vi "setCenter.vi"(8 "error in (no error)":errorcluster, 10 "center":T1, 11 "GObject in":refnum<class "GObject.lvclass">) -> (0 "error out":errorcluster, 3 "GObject out":refnum<class "GObject.lvclass">)   [LabVIEW 2023, in "TLC_Scripto.lvlib" / "GObject.lvclass"]
uses:
  GObject.lvclass
  GObject.lvclass/GObject.ctl
  Ctrls/point.ctl
  TLC_Scripto.lvlib
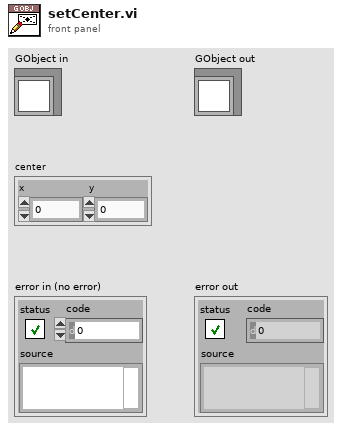
[diagram p1: front panel]
types:
  T1 = typedef "TLC_Scripto.lvlib/point.ctl" = cluster{"x":i32, "y":i32}
  T2 = typedef "TLC_Scripto.lvlib/rectangle.ctl" = cluster{"left":i32, "top":i32, "right":i32, "bottom":i32}
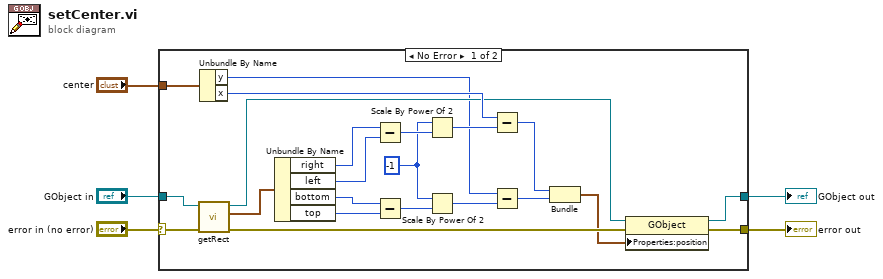
[diagram p0: block diagram]
diagram:
  n1 = case shown="No Error" "error in (no error)" {
    selector: "error in (no error)" -> [w27 w29]
    tunnel: [w15 w29] -> w4
    tunnel: [w17 w28] -> w2
    tunnel: "GObject in" -> [w26 w28]
    tunnel: "center" -> [w21 _]
    frame No Error {
      w9 = -1
      n2 = call-dynamic "getRect.vi"("error in (no error)"=w27, "GObject in"=w26) -> ("error out"=w16:errorcluster, "rectangle"=w25:T2, "GObject out"=w18:refnum<class "GObject.lvclass">)  [unwired: 7 in]
      n3 = Unbundle By Name(w21) -> ("y"=w8:i32, "x"=w20:i32)
      n4 = Unbundle By Name(w25) -> ("right"=w24:i32, "left"=w23:i32, "bottom"=w13:i32, "top"=w12:i32)
      n5 = Subtract(x=w24, y=w23) -> (x-y=w22:i32)
      n6 = Subtract(x=w13, y=w12) -> (x-y=w10:i32)
      n7 = Scale By Power Of 2(n=w9, x=w22) -> (x*2^n=w19:i32)
      n8 = Scale By Power Of 2(n=w9, x=w10) -> (x*2^n=w7:i32)
      n9 = Subtract(x=w20, y=w19) -> (x-y=w14:i32)
      n10 = Subtract(x=w8, y=w7) -> (x-y=w6:i32)
      n11 = Bundle(w14, w6) -> (w11:cluster{i32, i32})  [unwired: 1 in]
      n12 = property class="GObject"(reference=w18, error in=w16, "Properties:position"=w11) -> (reference out=w17:refnum<class "GObject.lvclass">, error out=w15:errorcluster)
    }
    frame Error {
    }
  }
  "error out" <- w4
  "GObject out" <- w2
